vi "_Pololu.Verification Test Util.vi"() -> ()   [LabVIEW 2018]
uses:
  <vilib>/KATE/Queues/Queue Utils.lvlib
  Dual Servo Manager Class/PololuCtrl.lvclass
  SubVIs/Pololu.Commands.ctl
  <vilib>/KATE/Module/Module Utils.lvlib
  <vilib>/KATE/Scheduler/Scheduler.lvlib
  <vilib>/KATE/Module/Module.SW Version Info.ctl
  <vilib>/KATE/Files/File Utils.lvlib
  <vilib>/KATE/Queues/Q.Element.ctl
  <vilib>/KATE/Module/Module.Working Dirs.ctl
  <vilib>/KATE/Module/Module Config.ctl
  SubVIs/Pololu.Device Range Config.ctl
  SubVIs/Pololu.Device Config.ctl
panel:
  in  "Tab Control":enum32{"Operate", "Maint"}(tab)
  in  "Store Lower Stop":bool
  in  "Store Upper Stop":bool
  in  "Pos Index":i32
  in  "Set Pos (Deg)":dbl(slide) max=270.0 scale=0.0..270.0 scale format="%.1f"
  out "Read Pos (us)":dbl max=270.0 format="%.1f"
  in  "Query Interval(s)":dbl=0.1
  in  "Query Status":bool
  out "Connected":bool
  out "error":errorcluster
  in  "Connect":bool
  in  "Disconnect":bool
  out "COM Port":string
  in  "Set Speed":bool
  in  "Set Accel":bool
  in  "us/10ms":dbl
  in  "us/10ms/80ms":dbl
  in  "Chan":u8
  in  "Set Pos":bool
  in  "Track Ctrl":bool
  out "Cmd us":dbl format="%.1f"
  out "Cmd units":u16
  in  "Store Pos":bool
  in  "Go To Pos":bool
  in  "Get Pos":bool
  out "Read Pos (Deg)":dbl max=270.0
  in  "Get Errors":bool
  out "Read Errors":u16 max=270 format="%016b"
  out "Moving":bool
  out "Config Dir":path
  in  "Module Config":T1={"Name"="DualServoCtrl", "Parent Q"=refnum, "Is Child?"=FALSE, "Index"=0, "Dirs"={"Root"=path "", "Config"=path "C:/ATE/Config", "Logs"=path "C:/ATE/Logs", "Reports"=path "C:/ATE/Reports", "App Data"=path "C:/ProgramData/MAIN"}, "Simulate"=FALSE, "SimCtrl"=refnum}
  in  "VID":string="1FFB"
  in  "PID":string="0089"
  out "Device Config":T3[](array[typedef])
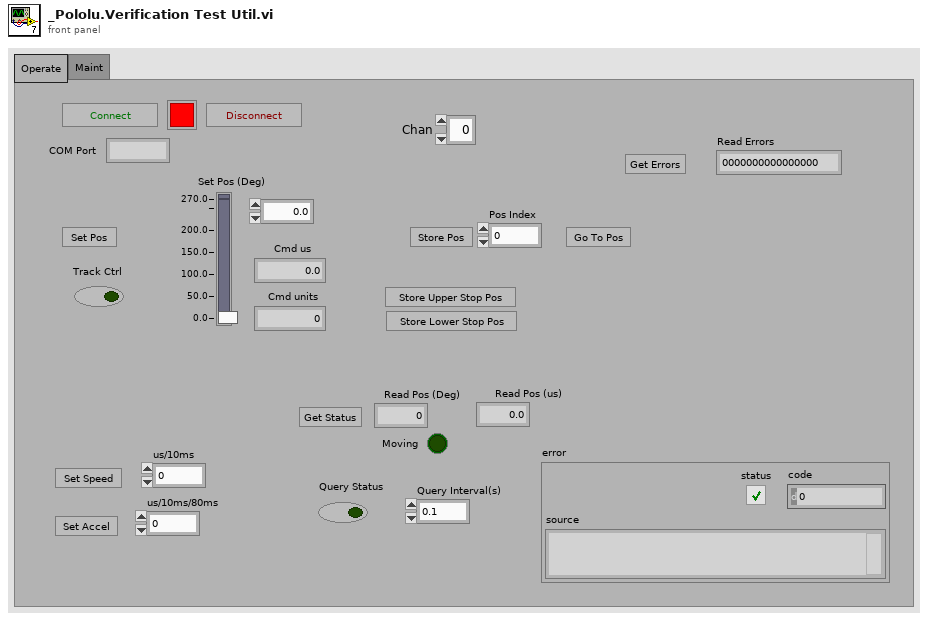
[diagram p1: front panel]
types:
  T1 = typedef "KATE_Lib.lvlib/Module Utils.lvlib/Module Config.ctl" = cluster{"Name":string, "Parent Q":refnum<queue>, "Is Child?":bool, "Index":i32, "Dirs":T2, "Simulate":bool, "SimCtrl":refnum<vi>}
  T2 = typedef "KATE_Lib.lvlib/Module Utils.lvlib/Module.Working Dirs.ctl" = cluster{"Root":path, "Config":path, "Logs":path, "Reports":path, "App Data":path}
  T3 = typedef "Pololu.Device Config.ctl" = cluster{"Chan":u8, "Accel":u16, "Speed":u16, "Positions":dbl[], "Range Info":T4}
  T4 = typedef "Pololu.Device Range Config.ctl" = cluster{"Min us":dbl, "Max us":dbl, "Min deg":dbl, "Max deg":dbl, "LStopDeg":dbl, "UStopDeg":dbl}
  T5 = typedef "KATE_Lib.lvlib/Module Utils.lvlib/Module.SW Version Info.ctl" = cluster{"AppName":string, "Company":string, "Version":string, "Description":string, "PN":string}
  T6 = typedef "KATE_Lib.lvlib/Module Utils.lvlib/Module Sys Info.ctl" = cluster{"Main Q":refnum<queue>, "Exe":bool, "SW Rev":T5, "Self Ref":refnum<vi>, "Main Tab":refnum<vi>, "Pane":refnum<vi>, "Stop":cluster{"Ref":refnum<event-registration>, "Event":refnum<user-event>}, "Cfg":T1, "Services":cluster{"Name":string, "vi ref":refnum<vi>}[], "Menu Ref":refnum<k9>, "CtrlStates":refnum<class "Class.SaveCtrls.lvclass">, "Docs":cluster{"Tags":string[], "Paths":path[]}, "Log":refnum<class "Event Notification.lvclass">, "Test Controls":refnum<vi>[], "Child Modules":cluster{"Name":string, "vi ref":refnum<vi>}[], "SW Items":string[][], "AppData":refnum<class "Class.AppData.lvclass">, "Subscriptions":refnum<class "Subscription.lvclass">}
  T7 = typedef "Pololu.Commands.ctl" = enum16{"Set Pos", "Set Speed", "Set Accel", "Get Pos", "Get Mov Status", "Get Errors"}
  T8 = cluster{"Pololu":refnum<class "PololuCtrl.lvclass">}
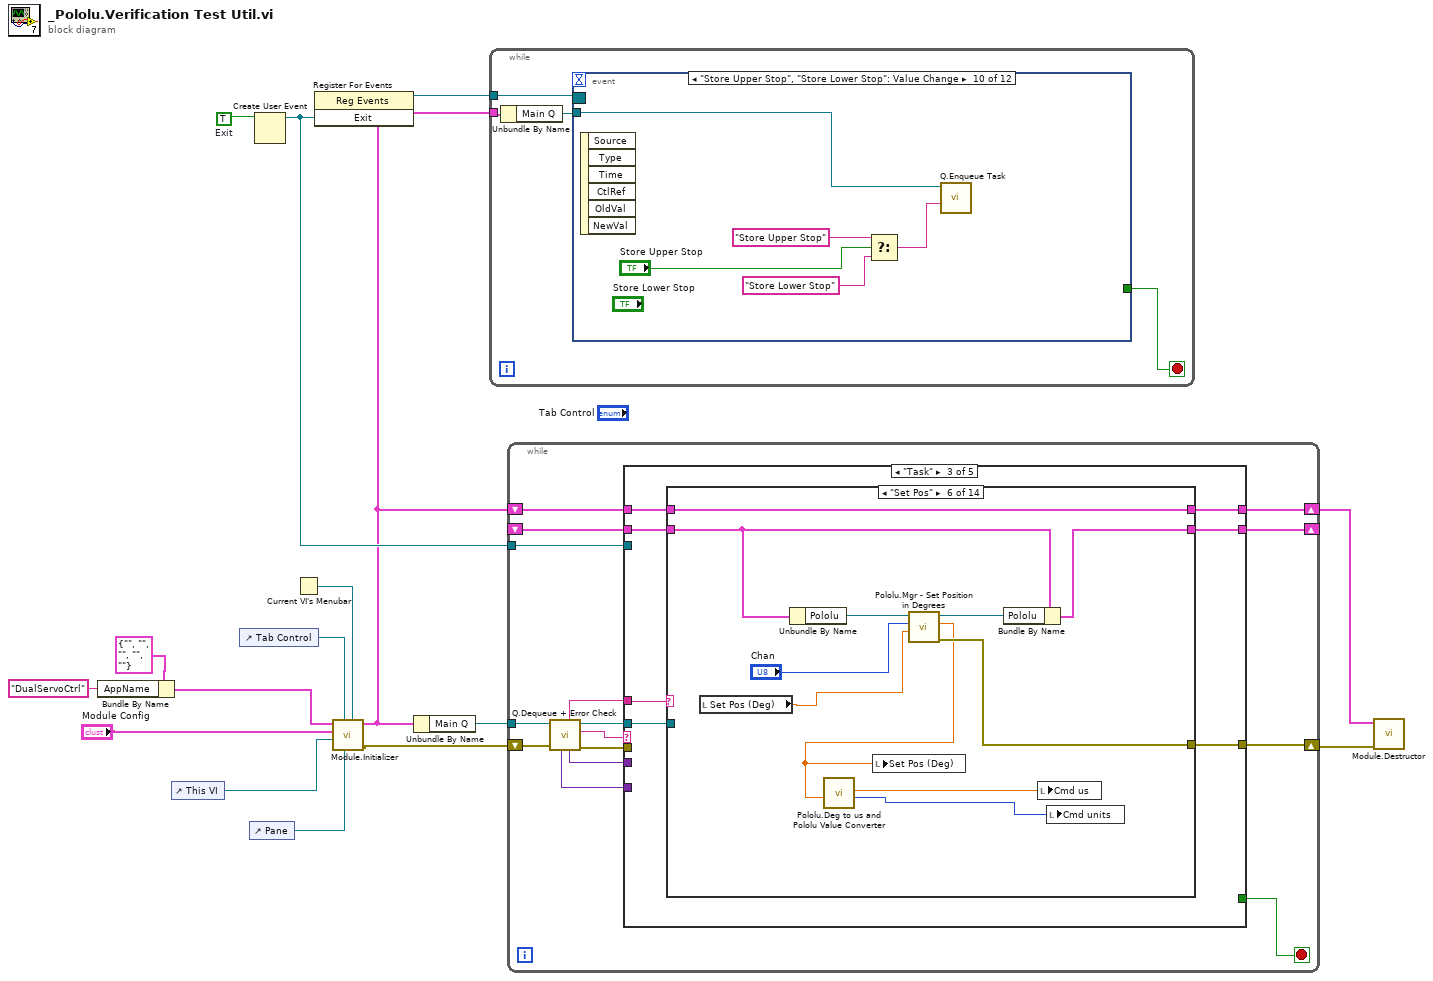
[diagram p0: block diagram]
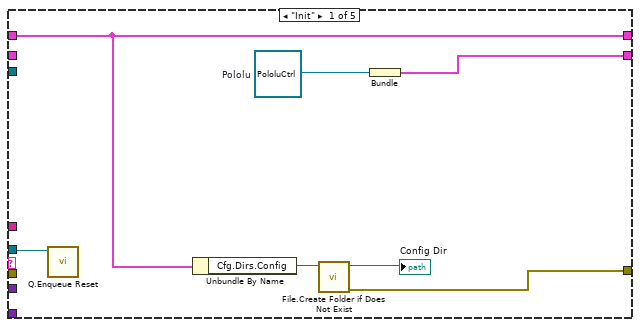
[diagram p2: hidden frame]
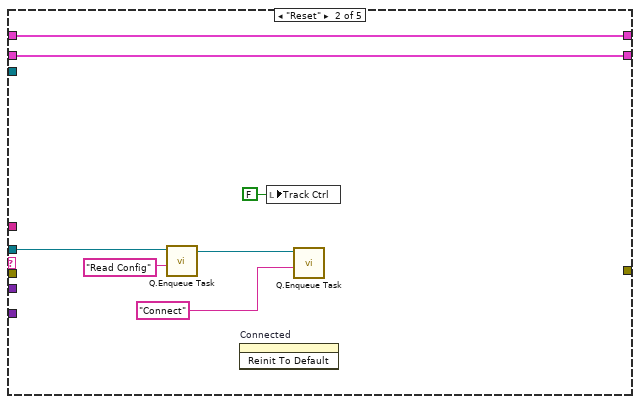
[diagram p3: hidden frame]
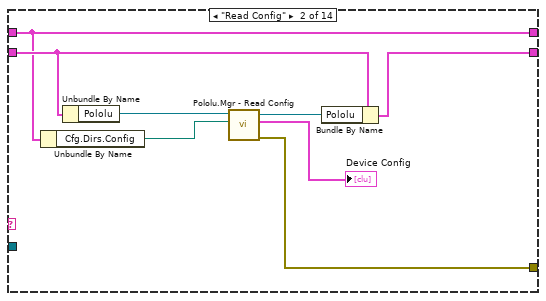
[diagram p5: hidden frame]
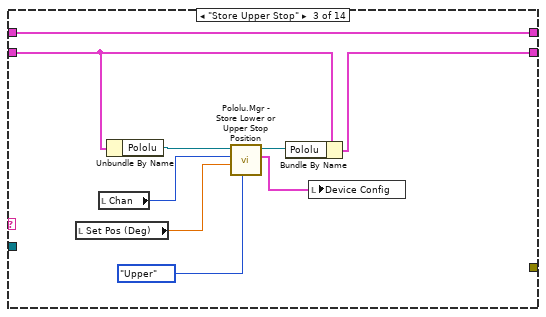
[diagram p6: hidden frame]
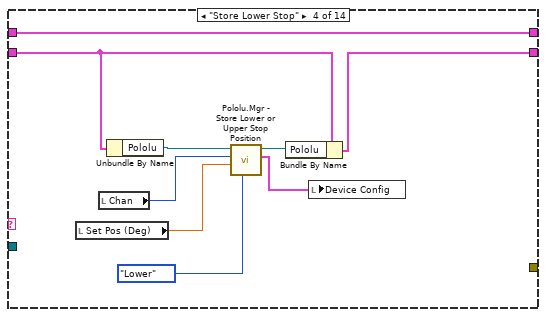
[diagram p7: hidden frame]
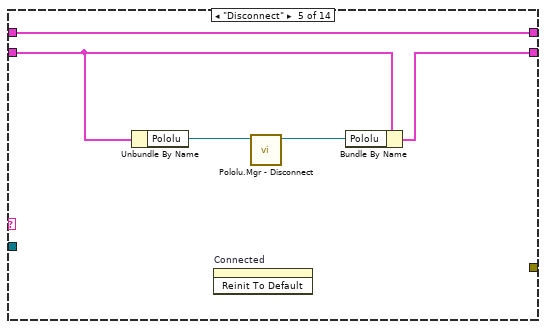
[diagram p8: hidden frame]
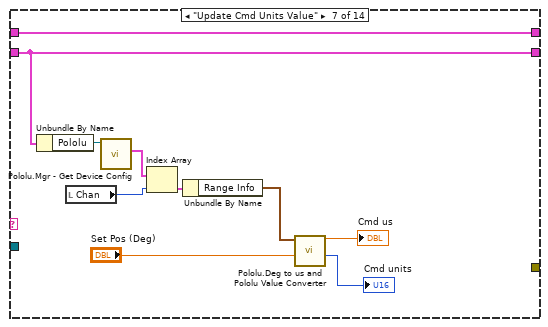
[diagram p9: hidden frame]
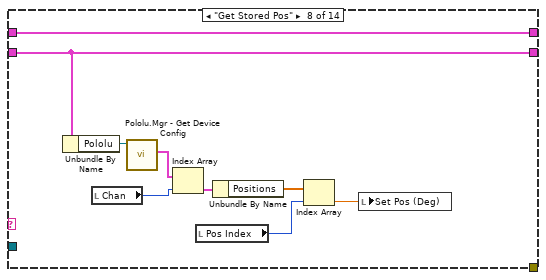
[diagram p10: hidden frame]
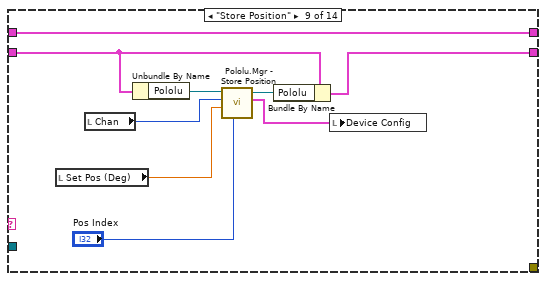
[diagram p11: hidden frame]
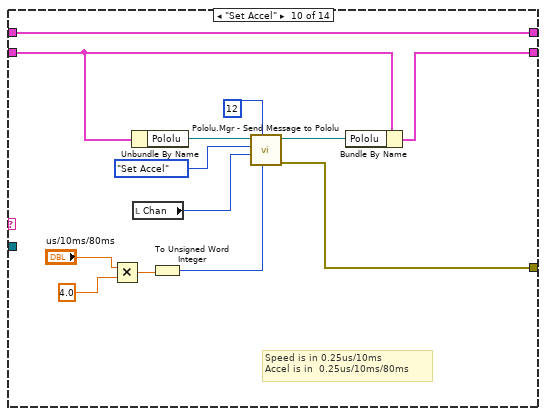
[diagram p12: hidden frame]
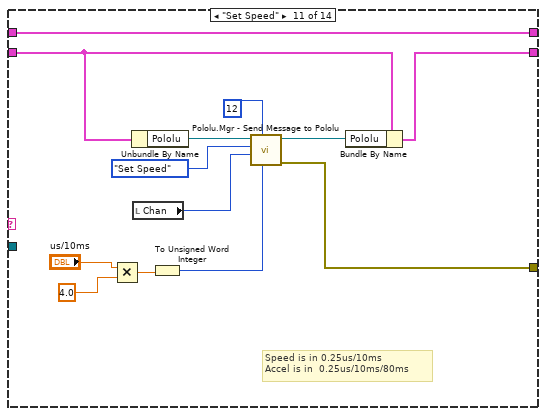
[diagram p13: hidden frame]
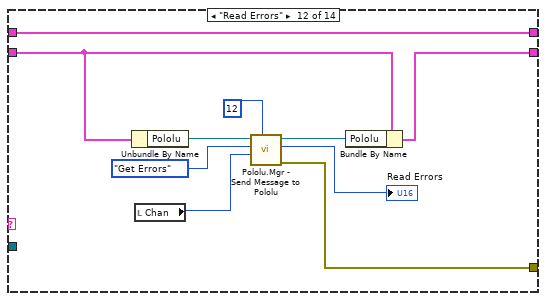
[diagram p14: hidden frame]
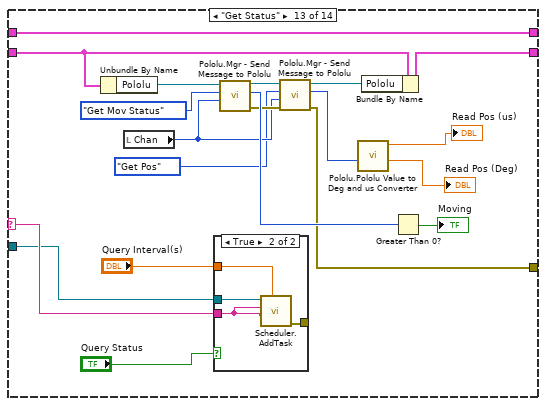
[diagram p15: hidden frame]
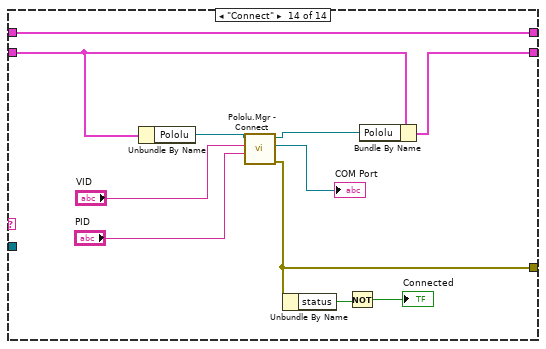
[diagram p17: hidden frame]
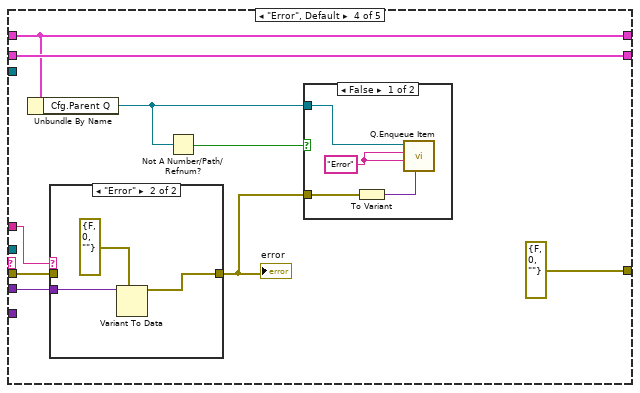
[diagram p18: hidden frame]
diagram:
  w16 = TRUE  # Exit
  n1 = Bundle By Name(cluster=T5 {"AppName"="", "Company"="", "Version"="", "Description"="", "PN"=""} ("SW Rev"), "AppName"="DualServoCtrl") -> (w5:T5)
  n2 = control-ref of="This VI"() -> (w10:refnum<vi>)
  n3 = control-ref of="Tab Control"() -> (w8:refnum<vi>)
  n4 = control-ref of="Pane"() -> (w7:refnum<vi>)
  n5 = Create User Event(user event datatype=w16) -> (user event=w15:refnum<user-event>)  [unwired: 1 in, 1 out]
  n6 = Current VI's Menubar() -> (w9:refnum<k9>)
  n7 = register-events(w15) -> (reference out=w14:refnum<event-registration>)  [unwired: 2 in, 1 out]
  n8 = call <vilib>:"Module.Initializer.vi"("Menu Ref"=w9, "Pane"=w7, "Main Tab"=w8, "Self Ref"=w10, "Module Config"="Module Config", "SW Rev"=w5) -> ("error out"=w13:errorcluster, "Sys"=w11:T6)  [unwired: 4 in]
  n9 = Unbundle By Name(w11) -> ("Main Q"=w12:refnum<queue>)
  n10 = while {
    tunnel: w11 -> [w17]
    tunnel: w14 -> [w20]
    stop <- w19 stop-if-true
    n11 = Unbundle By Name(w17) -> ("Main Q"=w18:refnum<queue>)
    n12 = event shown="[9] \"Store Upper Stop\", \"Store Lower Stop\": Value Change" {
      selector: w20 -> [_ _ _ _ _ _ _ _ _ _ _ _]
      dyn-events: _ -> [_ _ _ _ _ _ _ _ _ _ _ _]
      timeout: _ -> [_ _ _ _ _ _ _ _ _ _ _ _]
      tunnel: w18 -> [w25 w27 w29 w31 w32 w35 w41 w46 w49 w55 w57 w60]
      tunnel: [_ _ _ _ _ _ _ _ _ _ _ TRUE] -> w19
      event "Disconnect", "Connect": Value Change {
        n13 = event-data() -> ()  [unwired: 1 in, 6 out]
        n14 = Select(t="Connect", s="Connect", f="Disconnect") -> (s? t:f=w22:string)
        n15 = call <vilib>:"Q.Enqueue Task.vi"("Task Name"=w22, "Q In"=w25) -> ()  [unwired: 8 in, 2 out]
      }
      event "Set Pos": Value Change {
        n16 = event-data() -> ()  [unwired: 1 in, 6 out]
        n17 = call <vilib>:"Q.Enqueue Task.vi"("Task Name"="Set Pos", "Q In"=w27) -> ()  [unwired: 8 in, 2 out]
      }
      event "Set Speed": Value Change {
        n18 = event-data() -> ()  [unwired: 1 in, 6 out]
        n19 = call <vilib>:"Q.Enqueue Task.vi"("Task Name"="Set Speed", "Q In"=w29) -> ()  [unwired: 8 in, 2 out]
      }
      event "Set Accel": Value Change {
        n20 = event-data() -> ()  [unwired: 1 in, 6 out]
        n21 = call <vilib>:"Q.Enqueue Task.vi"("Task Name"="Set Accel", "Q In"=w31) -> ()  [unwired: 8 in, 2 out]
      }
      event "Get Pos": Value Change {
        n22 = event-data() -> ()  [unwired: 1 in, 6 out]
        n23 = call <vilib>:"Q.Enqueue Task.vi"("Task Name"="Get Status", "Q In"=w32) -> ()  [unwired: 8 in, 2 out]
      }
      event "Query Status": Value Change {
        n24 = event-data() -> ("NewVal"=w34:bool)  [unwired: 1 in, 5 out]
        n25 = case shown="True" w34 {
          tunnel: w35 -> [_ w39]
          frame False {
          }
          frame True {
            n26 = call <vilib>:"Q.Enqueue Task.vi"("Task Name"="Get Pos", "Q In"=w39) -> ("Q Out"=w36:refnum<queue>)  [unwired: 8 in, 1 out]
            n27 = call <vilib>:"Q.Enqueue Task.vi"("Task Name"="Get Status", "Q In"=w36) -> ()  [unwired: 8 in, 2 out]
          }
        }
      }
      event "Get Errors": Value Change {
        n28 = event-data() -> ()  [unwired: 1 in, 6 out]
        n29 = call <vilib>:"Q.Enqueue Task.vi"("Task Name"="Read Errors", "Q In"=w41) -> ()  [unwired: 8 in, 2 out]
      }
      event "Set Pos (Deg)": Value Change {
        n30 = event-data() -> ()  [unwired: 1 in, 6 out]
        n31 = Select(t="Set Pos", s="Track Ctrl", f="Update Cmd Units Value") -> (s? t:f=w44:string)
        n32 = call <vilib>:"Q.Enqueue Task.vi"("Task Name"=w44, "Q In"=w46) -> ()  [unwired: 8 in, 2 out]
      }
      event "Go To Pos": Value Change {
        n33 = event-data() -> ()  [unwired: 1 in, 6 out]
        n34 = call <vilib>:"Q.Enqueue Task.vi"("Task Name"="Get Stored Pos", "Q In"=w49) -> ("Q Out"=w47:refnum<queue>)  [unwired: 8 in, 1 out]
        n35 = call <vilib>:"Q.Enqueue Task.vi"("Task Name"="Set Pos", "Q In"=w47) -> ()  [unwired: 8 in, 2 out]
      }
      event "Store Upper Stop", "Store Lower Stop": Value Change {
        n36 = event-data() -> ()  [unwired: 1 in, 6 out]
        n37 = Select(t="Store Upper Stop" ("Task Name"), s="Store Upper Stop", f="Store Lower Stop" ("Task Name")) -> (s? t:f=w51:string)
        n38 = call <vilib>:"Q.Enqueue Task.vi"("Task Name"=w51, "Q In"=w55) -> ()  [unwired: 8 in, 2 out]
      }
      event "Store Pos": Value Change {
        n39 = event-data() -> ()  [unwired: 1 in, 6 out]
        n40 = call <vilib>:"Q.Enqueue Task.vi"("Task Name"="Store Position", "Q In"=w57) -> ()  [unwired: 8 in, 2 out]
      }
      event Panel Close? {
        n41 = event-data() -> ()  [unwired: 1 in, 4 out]
        n42 = call <vilib>:"Q.Enqueue Exit.vi"("Q In"=w60) -> ()  [unwired: 9 in, 2 out]
        n43 = event-data("Discard?"=TRUE) -> ()  [unwired: 1 in, 1 out]
      }
    }
  }
  n44 = while {
    tunnel: w12 -> [w75]
    shift-right: [w66] -> w4
    shift-left: w13 -> [w74]
    shift-right: [w64] -> _
    shift-left: _ -> [w68]
    tunnel: w15 -> [w63]
    shift-right: [w61] -> w3
    shift-left: w11 -> [w62]
    stop <- w65 stop-if-true
    n45 = call <vilib>:"Q.Dequeue + Error Check.vi"("Error In"=w74, "Q In"=w75) -> ("error out"=w67:errorcluster, "Cmd"=w73:string, "Q Out"=w72:refnum<queue>, "Data1"=w70:variant, "Sub"=w71:string, "Data2"=w69:variant)  [unwired: 4 in]
    n46 = case shown="\"Task\"" w73 {
      tunnel: w72 -> [w80 w87 w90 _ _]
      tunnel: w71 -> [_ _ w96 w240 _]
      tunnel: w70 -> [_ _ _ w247 _]
      tunnel: w69 -> [_ _ _ _ _]
      tunnel: w68 -> [_ w89 w95 w245 w260]
      tunnel: w67 -> [_ _ _ w248 _]
      tunnel: [w76 _ w93 errorcluster {"status"=FALSE, "code"=0, "source"=""} ("error") w257] -> w66
      tunnel: [_ _ _ _ TRUE] -> w65
      tunnel: [w81 w89 w94 w245 w260] -> w64
      tunnel: w63 -> [_ _ _ _ w262]
      tunnel: w62 -> [w79 w85 w92 w242 w259]
      tunnel: [w79 w85 w91 w242 w259] -> w61
      frame "Init" {
        w82 = refnum<class "PololuCtrl.lvclass"> refnum  # Pololu
        n47 = call <vilib>:"Q.Enqueue Reset.vi"("Q In"=w80) -> ()  [unwired: 9 in, 2 out]
        n48 = Unbundle By Name(w79) -> ("Cfg.Dirs.Config"=w78:path)
        n49 = call <vilib>:"File.Create Folder if Does Not Exist.vi"("Path"=w78) -> ("error out"=w76:errorcluster, "Dup Path"=→"Config Dir":path)  [unwired: 8 in, 1 out]
        n50 = Bundle("Pololu"=w82) -> (w81:T8)  [unwired: 1 in]
      }
      frame "Reset" {
        n51 = call <vilib>:"Q.Enqueue Task.vi"("Task Name"="Read Config", "Q In"=w87) -> ("Q Out"=w83:refnum<queue>)  [unwired: 8 in, 1 out]
        n52 = invoke on="Connected" class="Bool (strict)" method="Reinit To Default"() -> ()  [unwired: 3 in, 3 out]
        n53 = local write "Track Ctrl"(FALSE ("Track Ctrl")) -> ()
        n54 = call <vilib>:"Q.Enqueue Task.vi"("Task Name"="Connect", "Q In"=w83) -> ()  [unwired: 8 in, 2 out]
      }
      frame "Task" {
        n55 = case shown="\"Set Pos\"" w96 {
          selector: w96 -> [_ _ _ _ _ _ _ _ _ _ _ _ w215 _]
          tunnel: w95 -> [w98 w104 w112 w121 w129 w140 w149 w154 w164 w181 w194 w204 w224 w239]
          tunnel: [w98 w105 w113 w122 w128 w139 w149 w154 w165 w180 w193 w203 w223 w238] -> w94
          tunnel: [_ w102 _ _ _ w135 _ _ _ w175 w188 w198 w212 w232] -> w93
          tunnel: w92 -> [w97 w101 w115 w124 w125 w134 w150 w159 w168 w169 w182 w195 w218 w229]
          tunnel: [w97 w101 w115 w124 w125 w134 w150 w159 w168 w169 w182 w195 w218 w229] -> w91
          tunnel: w90 -> [_ _ _ _ _ _ _ _ _ _ _ _ w205 _]
          frame Default {
          }
          frame "Read Config" {
            n56 = Unbundle By Name(w101) -> ("Cfg.Dirs.Config"=w100:path)
            n57 = Unbundle By Name(w104) -> ("Pololu"=w106:refnum<class "PololuCtrl.lvclass">)
            n58 = call "Pololu.Mgr - Read Config.vi"("Config Folder"=w100, "PololuCtrl in"=w106) -> ("error out"=w102:errorcluster, "Devices"=→"Device Config":T3[], "PololuCtrl out"=w103:refnum<class "PololuCtrl.lvclass">)  [unwired: 7 in]
            n59 = Bundle By Name(cluster=w104, "Pololu"=w103) -> (w105:T8)
          }
          frame "Store Upper Stop" {
            n60 = local read "Set Pos (Deg)"() -> (w109:dbl)
            n61 = local read "Chan"() -> (w108:u8)
            n62 = Unbundle By Name(w112) -> ("Pololu"=w114:refnum<class "PololuCtrl.lvclass">)
            n63 = call "Pololu.Mgr - Store Lower or Upper Stop Position.vi"("Type"=enum16{"Lower", "Upper"}."Upper", "Pos(Deg)"=w109, "Channel"=w108, "PololuCtrl in"=w114) -> ("Device Config"=w110:T3[], "PololuCtrl out"=w111:refnum<class "PololuCtrl.lvclass">)  [unwired: 5 in, 1 out]
            n64 = Bundle By Name(cluster=w112, "Pololu"=w111) -> (w113:T8)
            n65 = local write "Device Config"(w110) -> ()
          }
          frame "Store Lower Stop" {
            n66 = local read "Set Pos (Deg)"() -> (w118:dbl)
            n67 = local read "Chan"() -> (w117:u8)
            n68 = Unbundle By Name(w121) -> ("Pololu"=w123:refnum<class "PololuCtrl.lvclass">)
            n69 = call "Pololu.Mgr - Store Lower or Upper Stop Position.vi"("Type"=enum16{"Lower", "Upper"}."Lower", "Pos(Deg)"=w118, "Channel"=w117, "PololuCtrl in"=w123) -> ("Device Config"=w119:T3[], "PololuCtrl out"=w120:refnum<class "PololuCtrl.lvclass">)  [unwired: 5 in, 1 out]
            n70 = Bundle By Name(cluster=w121, "Pololu"=w120) -> (w122:T8)
            n71 = local write "Device Config"(w119) -> ()
          }
          frame "Disconnect" {
            n72 = Unbundle By Name(w129) -> ("Pololu"=w127:refnum<class "PololuCtrl.lvclass">)
            n73 = invoke on="Connected" class="Bool (strict)" method="Reinit To Default"() -> ()  [unwired: 3 in, 3 out]
            n74 = call "Pololu.Mgr - Disconnect.vi"("PololuCtrl in"=w127) -> ("PololuCtrl out"=w126:refnum<class "PololuCtrl.lvclass">)  [unwired: 9 in, 1 out]
            n75 = Bundle By Name(cluster=w129, "Pololu"=w126) -> (w128:T8)
          }
          frame "Set Pos" {
            n76 = local read "Set Pos (Deg)"() -> (w131:dbl)
            n77 = Unbundle By Name(w140) -> ("Pololu"=w138:refnum<class "PololuCtrl.lvclass">)
            n78 = call "Pololu.Mgr - Set Position in Degrees.vi"("Pos(Deg)"=w131, "Channel"="Chan", "PololuCtrl in"=w138) -> ("error out"=w135:errorcluster, "Actual Pos(Deg)"=w130:dbl, "PololuCtrl out"=w137:refnum<class "PololuCtrl.lvclass">)  [unwired: 5 in, 1 out]
            n79 = call "Pololu.Deg to us and Pololu Value Converter.vi"("Set Pos (Deg)"=w130) -> ("Cmd units"=w132:u16, "Cmd us"=w133:dbl)  [unwired: 9 in]
            n80 = local write "Set Pos (Deg)"(w130) -> ()
            n81 = Bundle By Name(cluster=w140, "Pololu"=w137) -> (w139:T8)
            n82 = local write "Cmd us"(w133) -> ()
            n83 = local write "Cmd units"(w132) -> ()
          }
          frame "Update Cmd Units Value" {
            n84 = Unbundle By Name(w149) -> ("Pololu"=w148:refnum<class "PololuCtrl.lvclass">)
            n85 = local read "Chan"() -> (w146:u8)
            n86 = call "Pololu.Mgr - Get Device Config.vi"("PololuCtrl in"=w148) -> ("Device Config"=w147:T3[])  [unwired: 8 in, 2 out]
            n87 = Index Array(array=w147, index=w146) -> (element=w145:T3)
            n88 = Unbundle By Name(w145) -> ("Range Info"=w141:T4)
            n89 = call "Pololu.Deg to us and Pololu Value Converter.vi"("Set Pos (Deg)"="Set Pos (Deg)", "Range Info"=w141) -> ("Cmd units"=→"Cmd units":u16, "Cmd us"=→"Cmd us":dbl)  [unwired: 8 in]
          }
          frame "Get Stored Pos" {
            n90 = Unbundle By Name(w154) -> ("Pololu"=w158:refnum<class "PololuCtrl.lvclass">)
            n91 = local read "Chan"() -> (w156:u8)
            n92 = call "Pololu.Mgr - Get Device Config.vi"("PololuCtrl in"=w158) -> ("Device Config"=w157:T3[])  [unwired: 8 in, 2 out]
            n93 = Index Array(array=w157, index=w156) -> (element=w155:T3)
            n94 = local read "Pos Index"() -> (w152:i32)
            n95 = Unbundle By Name(w155) -> ("Positions"=w151:dbl[])
            n96 = Index Array(array=w151, index=w152) -> (element=w153:dbl)
            n97 = local write "Set Pos (Deg)"(w153) -> ()
          }
          frame "Store Position" {
            n98 = local read "Set Pos (Deg)"() -> (w162:dbl)
            n99 = local read "Chan"() -> (w163:u8)
            n100 = Unbundle By Name(w164) -> ("Pololu"=w167:refnum<class "PololuCtrl.lvclass">)
            n101 = call "Pololu.Mgr - Store Position.vi"("Index"="Pos Index", "Pos(Deg)"=w162, "Channel"=w163, "PololuCtrl in"=w167) -> ("Device Config"=w160:T3[], "PololuCtrl out"=w166:refnum<class "PololuCtrl.lvclass">)  [unwired: 5 in, 1 out]
            n102 = Bundle By Name(cluster=w164, "Pololu"=w166) -> (w165:T8)
            n103 = local write "Device Config"(w160) -> ()
          }
          frame "Set Accel" {
            # "Speed is in 0.25us/10ms\nAccel is in  0.25us/10ms/80ms"
            n104 = Multiply(x="us/10ms/80ms", y=4.0) -> (x*y=w172:dbl)
            n105 = Unbundle By Name(w181) -> ("Pololu"=w179:refnum<class "PololuCtrl.lvclass">)
            n106 = local read "Chan"() -> (w174:u8)
            n107 = To Unsigned Word Integer(number=w172) -> (unsigned 16bit integer=w171:u16)
            n108 = call "Pololu.Mgr - Send Message to Pololu.vi"("Value"=w171, 7:u8 12 ("Device"), "Channel"=w174, "Command"=Pololu.Commands."Set Accel", "PololuCtrl in"=w179) -> ("error out"=w175:errorcluster, "PololuCtrl out"=w178:refnum<class "PololuCtrl.lvclass">)  [unwired: 4 in, 1 out]
            n109 = Bundle By Name(cluster=w181, "Pololu"=w178) -> (w180:T8)
          }
          frame "Set Speed" {
            # "Speed is in 0.25us/10ms\nAccel is in  0.25us/10ms/80ms"
            n110 = Multiply(x="us/10ms", y=4.0) -> (x*y=w185:dbl)
            n111 = Unbundle By Name(w194) -> ("Pololu"=w192:refnum<class "PololuCtrl.lvclass">)
            n112 = local read "Chan"() -> (w187:u8)
            n113 = To Unsigned Word Integer(number=w185) -> (unsigned 16bit integer=w184:u16)
            n114 = call "Pololu.Mgr - Send Message to Pololu.vi"("Value"=w184, 7:u8 12 ("Device"), "Channel"=w187, "Command"=Pololu.Commands."Set Speed", "PololuCtrl in"=w192) -> ("error out"=w188:errorcluster, "PololuCtrl out"=w191:refnum<class "PololuCtrl.lvclass">)  [unwired: 4 in, 1 out]
            n115 = Bundle By Name(cluster=w194, "Pololu"=w191) -> (w193:T8)
          }
          frame "Read Errors" {
            n116 = Unbundle By Name(w204) -> ("Pololu"=w202:refnum<class "PololuCtrl.lvclass">)
            n117 = local read "Chan"() -> (w197:u8)
            n118 = call "Pololu.Mgr - Send Message to Pololu.vi"(7:u8 12 ("Device"), "Channel"=w197, "Command"=Pololu.Commands."Get Errors", "PololuCtrl in"=w202) -> ("error out"=w198:errorcluster, "Response"=→"Read Errors":u16, "PololuCtrl out"=w201:refnum<class "PololuCtrl.lvclass">)  [unwired: 5 in]
            n119 = Bundle By Name(cluster=w204, "Pololu"=w201) -> (w203:T8)
          }
          frame "Get Status" {
            n120 = Unbundle By Name(w224) -> ("Pololu"=w222:refnum<class "PololuCtrl.lvclass">)
            n121 = local read "Chan"() -> (w210:u8)
            n122 = case shown="True" "Query Status" {
              tunnel: w205 -> [_ w228]
              tunnel: "Query Interval(s)" -> [_ w227]
              tunnel: w215 -> [_ w225]
              tunnel: [_ w226] -> _
              frame False {
              }
              frame True {
                n123 = call <vilib>:"Scheduler.AddTask.vi"("Interval(s)"=w227, "Task Name"=w225, "Sched Name"=w225, "Q In"=w228) -> ("Error Out"=w226:errorcluster)  [unwired: 6 in, 1 out]
              }
            }
            n124 = call "Pololu.Mgr - Send Message to Pololu.vi"("Channel"=w210, "Command"=Pololu.Commands."Get Mov Status", "PololuCtrl in"=w222) -> ("error out"=w213:errorcluster, "Response"=w220:u16, "PololuCtrl out"=w214:refnum<class "PololuCtrl.lvclass">)  [unwired: 6 in]
            n125 = call "Pololu.Mgr - Send Message to Pololu.vi"("error in (no error)"=w213, "Channel"=w210, "Command"=Pololu.Commands."Get Pos", "PololuCtrl in"=w214) -> ("error out"=w212:errorcluster, "Response"=w206:u16, "PololuCtrl out"=w211:refnum<class "PololuCtrl.lvclass">)  [unwired: 5 in]
            n126 = call "Pololu.Pololu Value to Deg and us Converter.vi"("Pololu Value"=w206) -> ("Pos (Deg)"=→"Read Pos (Deg)":dbl, "Pos (us)"=→"Read Pos (us)":dbl)  [unwired: 9 in]
            n127 = Bundle By Name(cluster=w224, "Pololu"=w211) -> (w223:T8)
            n128 = Greater Than 0?(x=w220) -> (x > 0?=→"Moving":bool)
          }
          frame "Connect" {
            n129 = Unbundle By Name(w239) -> ("Pololu"=w237:refnum<class "PololuCtrl.lvclass">)
            n130 = call "Pololu.Mgr - Connect.vi"("PID"="PID", "VID"="VID", "PololuCtrl in"=w237) -> ("error out"=w232:errorcluster, "Com Port"=→"COM Port":refnum<visa-resource-name>, "PololuCtrl out"=w236:refnum<class "PololuCtrl.lvclass">)  [unwired: 6 in]
            n131 = Unbundle By Name(w232) -> ("status"=w231:bool)
            n132 = Not(x=w231) -> (.not. x?=→"Connected":bool)
            n133 = Bundle By Name(cluster=w239, "Pololu"=w236) -> (w238:T8)
          }
        }
      }
      frame "Error", Default {
        n134 = Unbundle By Name(w242) -> ("Cfg.Parent Q"=w241:refnum<queue>)
        n135 = case shown="\"Error\"" w240 {
          tunnel: w248 -> [w253 _]
          tunnel: [w253 w255] -> w243
          tunnel: w247 -> [_ w256]
          frame Default {
          }
          frame "Error" {
            n136 = Variant To Data(type=errorcluster {"status"=FALSE, "code"=0, "source"=""} ("error"), Variant=w256) -> (data=w255:errorcluster)  [unwired: 1 in, 1 out]
          }
        }
        "error" <- w243
        n137 = Not A Number/Path/Refnum?(number/path/refnum=w241) -> (NaN/Path/Refnum?=w244:bool)
        n138 = case shown="False" w244 {
          tunnel: w241 -> [w252 _]
          tunnel: w243 -> [w249 _]
          frame False {
            w251 = "Error" ("Cmd")
            n139 = To Variant(anything=w249) -> (Variant=w250:variant)
            n140 = call <vilib>:"Q.Enqueue Item.vi"("Data1"=w250, "Sub"=w251, "Cmd"=w251, "Q In"=w252) -> ()  [unwired: 6 in, 2 out]
          }
          frame True {
          }
        }
      }
      frame "Exit" {
        n141 = Generate User Event(user event=w262, event data cluster=TRUE) -> ()  [unwired: 2 in, 2 out]
        n142 = invoke on="Connected" class="Bool (strict)" method="Reinit To Default"() -> ()  [unwired: 3 in, 3 out]
        n143 = Unbundle By Name(w260) -> ("Pololu"=w261:refnum<class "PololuCtrl.lvclass">)
        n144 = call "Pololu.Mgr - Disconnect.vi"("PololuCtrl in"=w261) -> ("PololuCtrl out"=w258:refnum<class "PololuCtrl.lvclass">)  [unwired: 9 in, 1 out]
        n145 = call "Pololu.Mgr - Save Config.vi"("PololuCtrl in"=w258) -> ("error out"=w257:errorcluster)  [unwired: 9 in, 1 out]
      }
    }
  }
  n146 = call <vilib>:"Module.Destructor.vi"("error in"=w4, "Sys"=w3) -> ()  [unwired: 9 in, 1 out]
